vi "AppendToOutput.vi"(3 "error in":errorcluster, 4 "Input String":string, 5 "Output Refnum In":refnum<vi>) -> (0 "error out":errorcluster, 2 "Output Refnum Out":refnum<vi>)   [LabVIEW 2022 SP3]
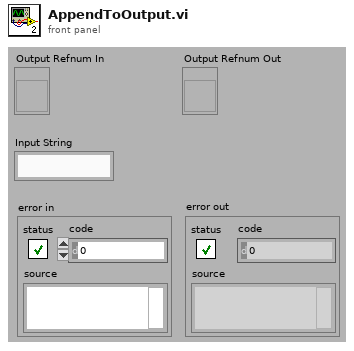
[diagram p1: front panel]
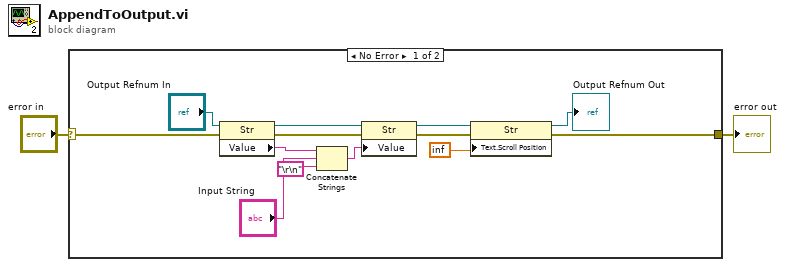
[diagram p0: block diagram]
diagram:
  n1 = case shown="No Error" "error in" {
    selector: "error in" -> [w8 w16]
    tunnel: [w3 w16] -> w2
    frame No Error {
      n2 = property on="Property Node" class="Str"(reference="Output Refnum In", error in=w8) -> (reference out=w10:refnum<vi>, error out=w9:errorcluster, "Value"=w13:string)
      n3 = Concatenate Strings(w13, "Input String", "\r\n") -> (w12:string)
      n4 = property class="Str"(reference=w10, error in=w9, "Value"=w12) -> (reference out=w7:refnum<vi>, error out=w6:errorcluster)
      n5 = property class="Str"(reference=w7, error in=w6, "Text.Scroll Position"=inf) -> (reference out=→"Output Refnum Out":refnum<vi>, error out=w3:errorcluster)
    }
    frame Error {
    }
  }
  "error out" <- w2
